vi "AlazarQueryCapability.vi"(0 "Handle":u64, 1 "Capability":u32(ring) items=["Get Serial Number"=268435492, "Get Latest Cal. Date"=268435494, "Get Latest Cal. Month"=268435501, "Get Latest Cal. Day"=268435502, "Get Latest Cal. Year"=268435503, "Memory Size"=268435498, "Board Type"=268435499, "ASOPC Type"=268435500, "Get PCIe Link Speed "=268435504, "Get PCIe Link Width"=268435505, "Get Max Pretrigger Samples"=268435526, "Get CPF Device"=268435569], 2 "error in (no error)":errorcluster) -> (3 "Handle":u64, 4 "Value":u32, 5 "Return Code":u32, 6 "error out":errorcluster)   [LabVIEW 2018]
doc: "Get a device attribute."
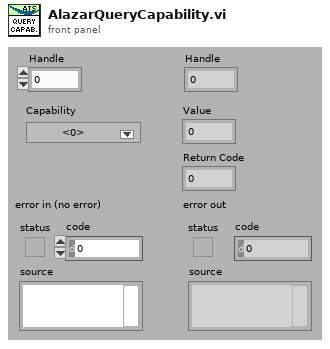
[diagram p1: front panel]
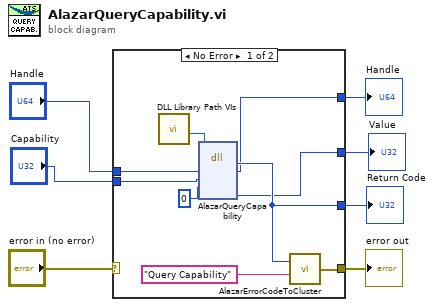
[diagram p0: block diagram]
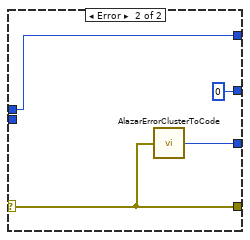
[diagram p2: hidden frame]
diagram:
  n1 = case shown="No Error" "error in (no error)" {
    selector: "error in (no error)" -> [_ w20]
    tunnel: [w13 w20] -> w6
    tunnel: [w15 w19] -> w5
    tunnel: "Handle" -> [w16 w18]
    tunnel: [w12 w18] -> w3
    tunnel: "Capability" -> [w11 _]
    tunnel: [w10 0] -> w1
    frame No Error {
      n2 = call "DLL Library Path VIs.vi"() -> ("Alazar"=w8:path)  [unwired: 9 in, 2 out]
      n3 = dll-call lib="C:/Project/SerialSectOCT - FFT GPU/SerialSectOCT/Labview Software/DLL/ATSApi.dll" fn="AlazarQueryCapability"(path in=w8, "handle"=w16, "capability"=w11, "reserved"=u32 0) -> ("return type"=w15:u32, "handle"=w12:u64, "value"=w10:u32)  [unwired: 5 in, 2 out]
      n4 = call "AlazarErrorCodeToCluster.vi"("Message"="Query Capability", "Error Code"=w15) -> ("error out"=w13:errorcluster)
    }
    frame Error {
      n5 = call "AlazarErrorClusterToCode.vi"("error in (no error)"=w20) -> ("Error Code"=w19:u32)
    }
  }
  "Handle" <- w3
  "error out" <- w6
  "Return Code" <- w5
  "Value" <- w1
